vi "Create Events.vi"(8 "error in (no error)":errorcluster, 11 "New Server in":T1 caption="New Server") -> (0 "error out":errorcluster, 3 "New Server out":T1 caption="New Server")   [LabVIEW 2025, in "MCP Server.lvlib"]
uses:
  MCP Server.lvlib
  Server Data.ctl
  <vilib>/IlluminatedG/IG HTTP Server/HTTP Server/Server/Server.lvclass
  Tool Data.ctl
  Input Parameter.ctl
  Output Parameter.ctl
  Logging.ctl
  User Events.ctl
  onRpc.ctl
  Prompt Data.ctl
  Prompt Argument.ctl
  resource data.ctl
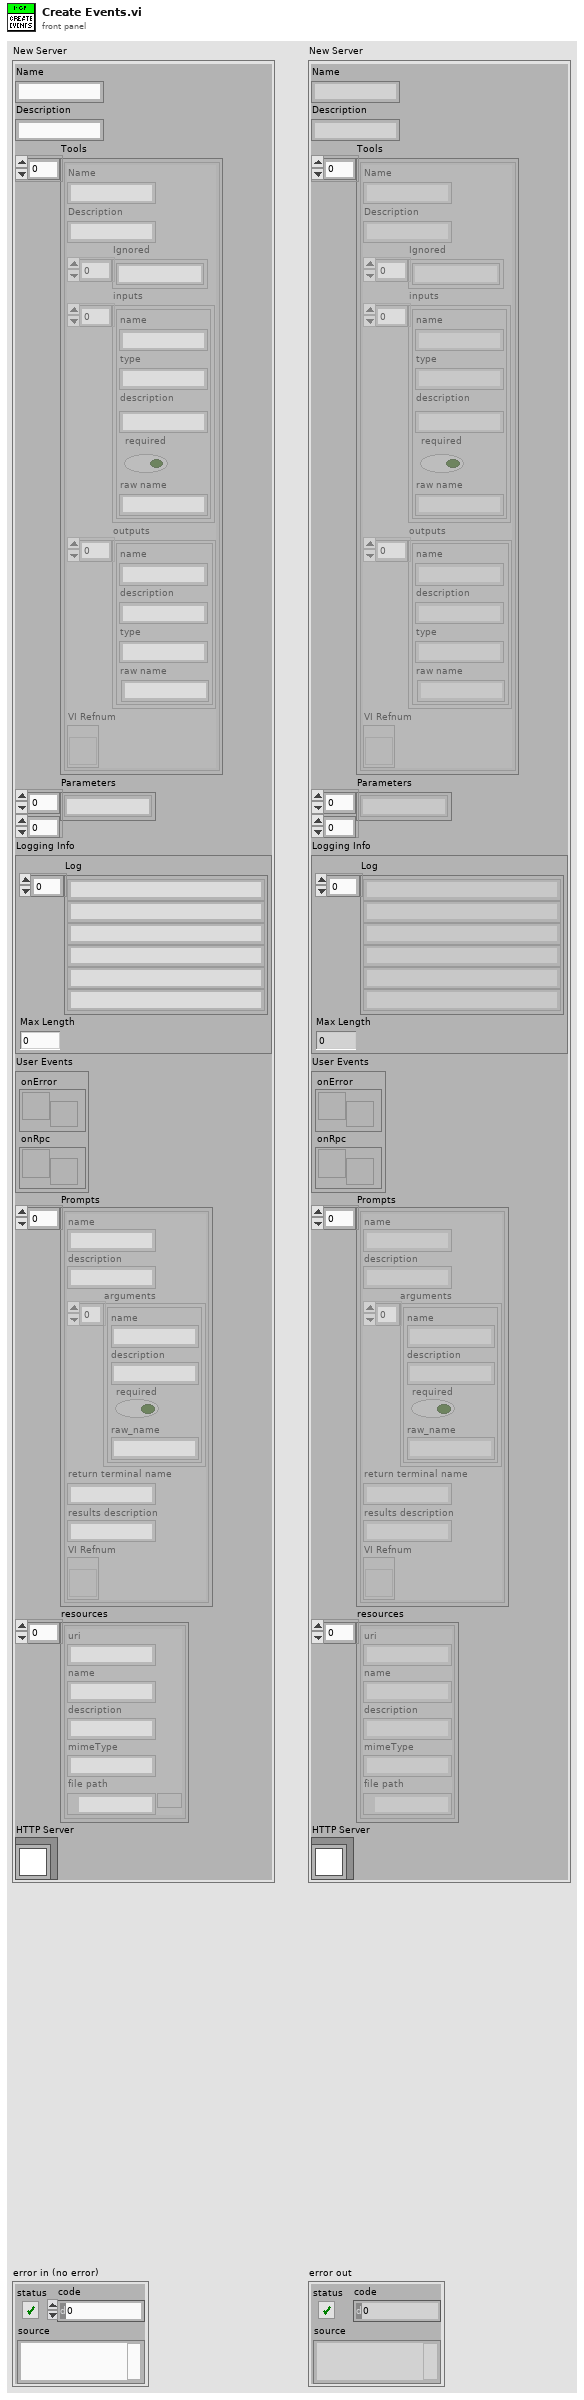
[diagram p1: front panel]
types:
  T1 = typedef "MCP Server.lvlib/Server Data.ctl" = cluster{"Name":string, "Description":string, "Tools":T2[], "Parameters":string[][], "Logging Info":T5, "User Events":T6, "Prompts":T7[], "resources":T9[], "HTTP Server":refnum<class "Server.lvclass">}
  T2 = typedef "MCP Server.lvlib/Tool Data.ctl" = cluster{"Name":string, "Description":string, "Ignored":string[], "inputs":T3[], "outputs":T4[], "VI Refnum":refnum<vi>}
  T3 = typedef "MCP Server.lvlib/Input Parameter.ctl" = cluster{"name":string, "type":string, "description":string, "required":bool, "raw name":string}
  T4 = typedef "MCP Server.lvlib/Output Parameter.ctl" = cluster{"name":string, "description":string, "type":string, "raw name":string}
  T5 = typedef "MCP Server.lvlib/Logging.ctl" = cluster{"Log":string[], "Max Length":i32}
  T6 = typedef "MCP Server.lvlib/User Events.ctl" = cluster{"onError":refnum<user-event>, "onRpc":refnum<user-event>}
  T7 = typedef "MCP Server.lvlib/Prompt Data.ctl" = cluster{"name":string, "description":string, "arguments":T8[], "return terminal name":string, "results description":string, "VI Refnum":refnum<vi>}
  T8 = typedef "MCP Server.lvlib/Prompt Argument.ctl" = cluster{"name":string, "description":string, "required":bool, "raw_name":string}
  T9 = typedef "MCP Server.lvlib/resource data.ctl" = cluster{"uri":string, "name":string, "description":string, "mimeType":string, "file path":path}
  T10 = typedef "MCP Server.lvlib/onRpc.ctl" = cluster{"request":string, "response":string}
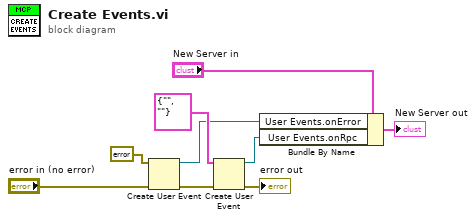
[diagram p0: block diagram]
diagram:
  n1 = Create User Event(user event datatype=errorcluster {"status"=FALSE, "code"=0, "source"=""} ("error constant"), error in="error in (no error)") -> (user event=w1:refnum<user-event>, error out=w3:errorcluster)
  n2 = Create User Event(user event datatype=T10 {"request"="", "response"=""} ("onRpc"), error in=w3) -> (user event=w9:refnum<user-event>, error out=→"error out":errorcluster)
  n3 = Bundle By Name(cluster="New Server in", "User Events.onError"=w1, "User Events.onRpc"=w9) -> (→"New Server out":T1)
